vi "Set Endpoint Configuration Property.vi"(8 "error in":errorcluster, 9 "configuration":T2, 10 "endpoint":string, 11 "endpoint configuration in":T1 format="%.0x") -> (0 "error out":errorcluster, 3 "endpoint configuration out":T1 format="%.0x")   [LabVIEW 2019, in "SLSC Switch Scripting.lvlib"]
uses:
  SLSC Switch Scripting.lvlib
  <vilib>/NI VeriStand/Custom Device API/Custom Device Item Ref.ctl
  Shared/Endpoint Configuration Enum.ctl
  <vilib>/NI VeriStand/Custom Device API/Set Item Property (String).vi
  <vilib>/NI VeriStand/Custom Device API/Custom Device API.lvlib
  Shared/SLSC Switch Shared.lvlib
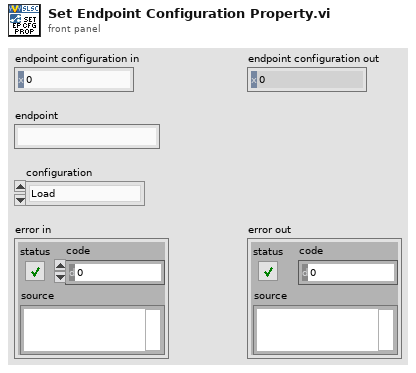
[diagram p1: front panel]
types:
  T1 = typedef "Custom Device API.lvlib/Custom Device Item Ref.ctl" = u64
  T2 = typedef "SLSC Switch Shared.lvlib/Endpoint Configuration Enum.ctl" = enum16{"Load", "Source", "Configuration"}
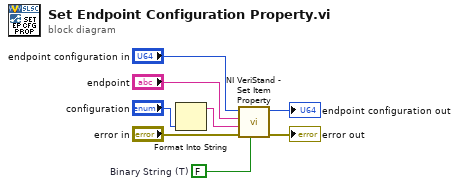
[diagram p0: block diagram]
diagram:
  w3 = FALSE  # Binary String (T)
  n1 = Format Into String("configuration") -> (resulting string=w6:string)  [unwired: 3 in, 1 out]
  n2 = call-poly <vilib>:"NI VeriStand - Set Item Property.vi"("Binary String (T)"=w3, "error in (no error)"="error in", "Value"=w6, "Property Name"="endpoint", "Item Ref in"="endpoint configuration in") -> ("error out"=→"error out":errorcluster, "Item Ref out"=→"endpoint configuration out":T1)  [unwired: 4 in, 1 out]
